vi "combined_broken.vi"() -> ()   [LabVIEW 2020]
uses:
  C:/Users/Public/Documents/Photometrics/PMQI-LabViewSamples/Examples/2018/Dependencies/PVCamNET.dll
  Dependencies/PVCamNET.dll
panel:
  out "SavingPath":string
  out "Saving":bool
  out "Capturing":bool
  in  "seq_save":bool
  in  "seq_start":bool
  in  "Path":path
  in  "FramesToCapture":u16=10
  in  "Full CCD Height":u16
  in  "Full CCD Width":u16
  in  "Full CCD":bool
  in  "Get ROI":bool
  in  "Height":u16
  in  "Y":u16
  in  "Width":u16
  in  "X":u16
  out "Trigger Mode":i32
  in  "Trigger In Behaviour":string(combo)="Edge Trigger"
  out "Exp. out":i32
  in  "Trigger Out Behaviour":string(combo)="Any Row"
  out "Boolean":bool
  in  "Scan Direction Reset":bool
  out "Scan Line Time":dbl format="%#_14g"
  in  "Scan Width":dbl=16.0
  in  "Scan Line Delay":dbl
  in  "Scan Direction":string(combo)="Up"
  in  "Scan Mode":string(combo)="Scan Width"
  in  "Exposure Time":dbl=5.0
  in  "Live":bool
  in  "Camera Status":bool
  in  "Uninit":bool
  in  "Live stop":bool
  in  "Live start":bool
  in  "Open":bool
  # "Description:\nThis interface can be used for both live imaging\nand sequence acquisition.\n\nSteps to run:\n1. Click the \"Run\" arrow\n2. Click \"Open\"\n3. Add desired parameters\n\nTo run live imaging: click \"Live Start\". If\nparameters need to be changed while imaging,\nfirst click \"Live Stop\" and then change\nparameters before starting again.\n\nTo execute sequence acquisition: click\n\"Sequence Start\". AFTER sequence has been\ncompleted (signified by the \"Capturing\" light\nturning off), click \"Sequence Save\" to save\nimages to desired folder.\n\n4. Click \"Close\" after finished imaging"
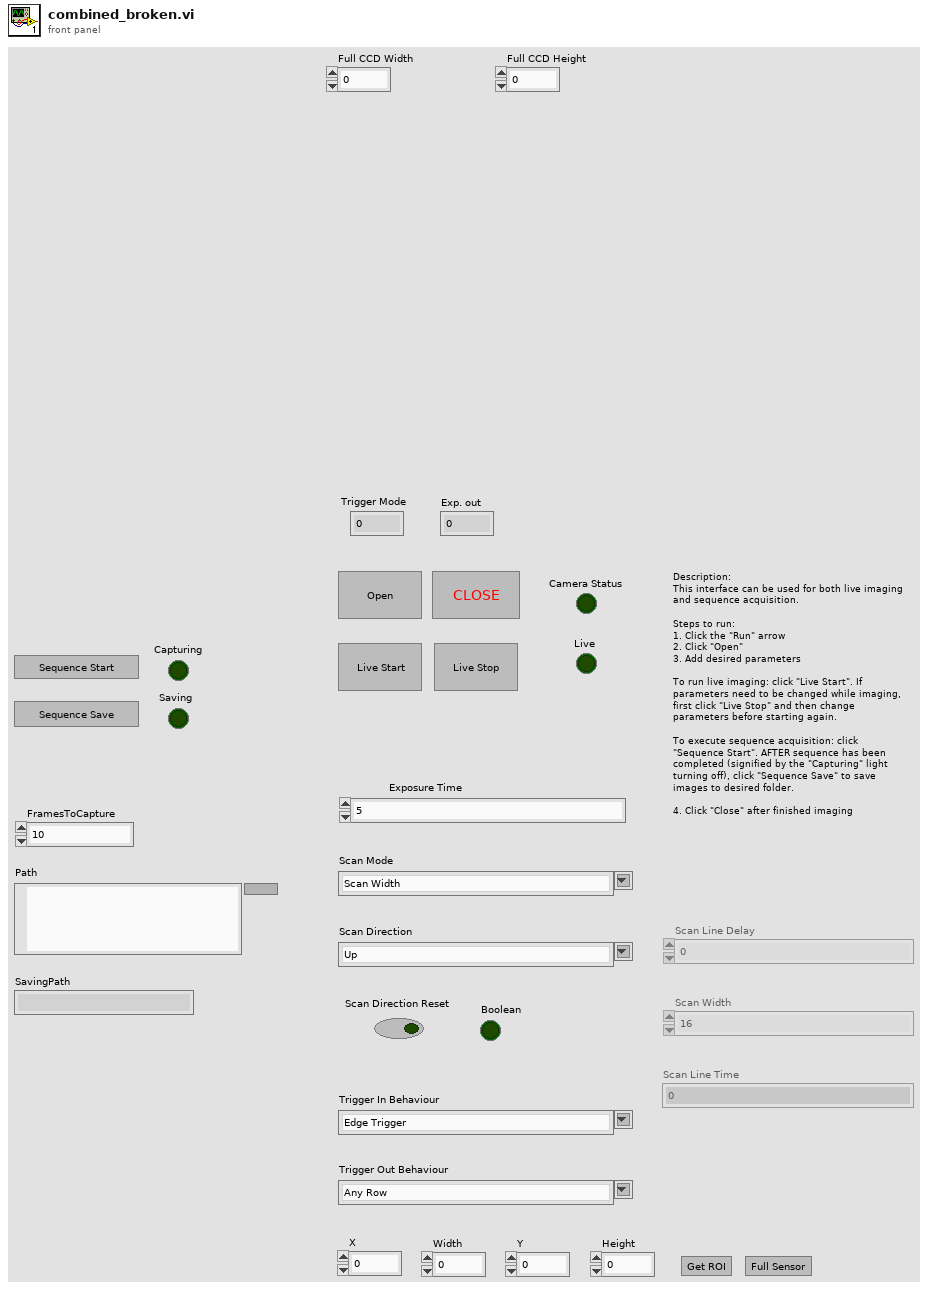
[diagram p1: front panel]
types:
  T1 = enum8{"Enabled", "Disabled", "Disabled and Grayed Out"}
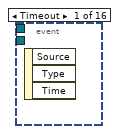
[diagram p2: hidden frame]
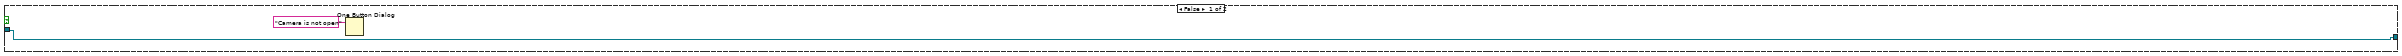
[diagram p15: hidden frame]
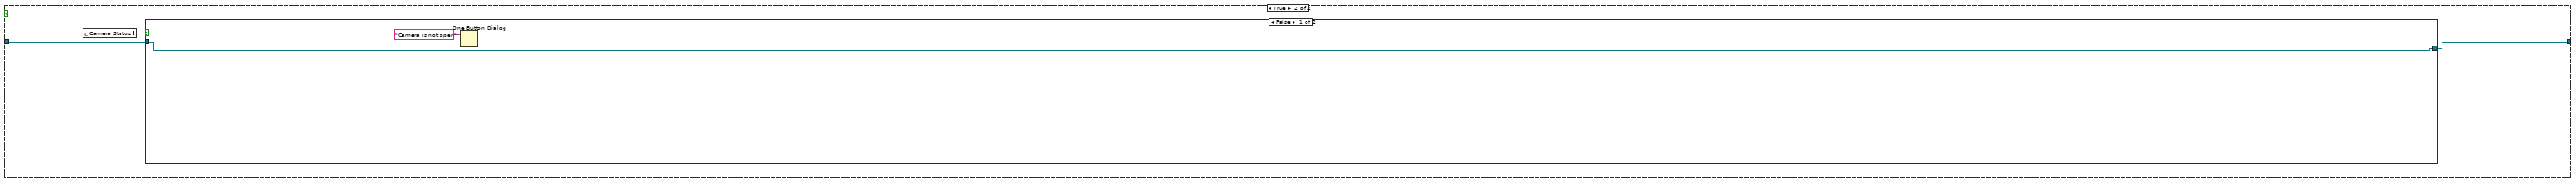
[diagram p18: hidden frame]
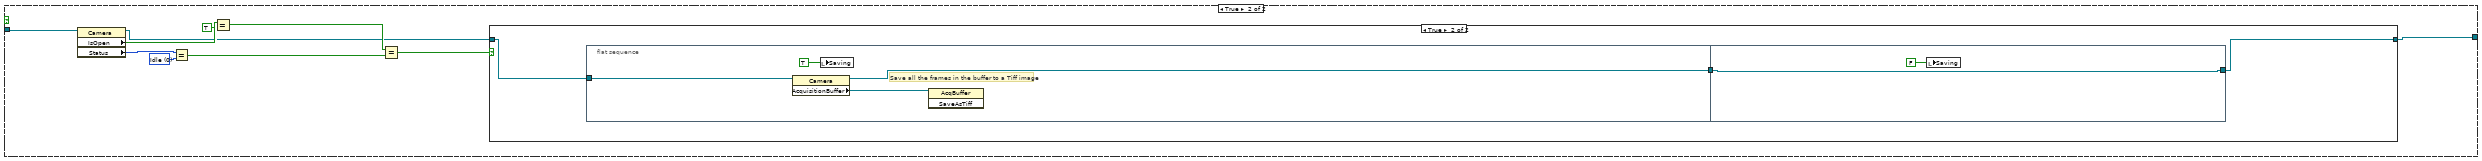
[diagram p19: hidden frame]
diagram:
  w16 = T1."Disabled and Grayed Out" ("Disabled")
  n1 = flat-sequence {
    tunnel: [w32] -> w31
    tunnel: w31 -> [w34]
    tunnel: [w33] -> w30
    tunnel: w30 -> [w874]
    frame #0 {
      n2 = property class="Library"() -> ("Instance"=w32:refnum<k24>)  [unwired: 2 in, 2 out]
    }
    frame #1 {
      n3 = while {
        tunnel: w34 -> [w39]
        shift-right: [w38] -> _
        shift-left: _ -> [w36]
        tunnel: [w37] -> w33
        stop <- w35 stop-if-true
        n4 = event shown="[1] \"Open\": Value Change" {
          selector: _ -> [_ _ _ _ _ _ _ _ _ _ _ _ _ _ _ _]
          dyn-events: _ -> [_ _ _ _ _ _ _ _ _ _ _ _ _ _ _ _]
          timeout: _ -> [_ _ _ _ _ _ _ _ _ _ _ _ _ _ _ _]
          tunnel: w39 -> [_ w44 _ _ _ _ _ _ w548 _ _ _ _ w791 _ w846]
          tunnel: [_ w43 w203 w234 w261 w293 w425 w489 w549 w616 w653 w726 w753 w792 w821 w847] -> w38
          tunnel: [_ w42 _ _ _ _ _ _ w548 _ _ _ _ w791 _ w846] -> w37
          tunnel: w36 -> [_ w41 w204 w233 w265 w294 w431 w491 w550 w617 w654 w727 w754 w793 w822 w848]
          tunnel: [_ _ _ _ _ _ _ _ _ _ _ _ _ _ _ w845] -> w35
          event Timeout {
            n5 = event-data() -> ()  [unwired: 1 in, 3 out]
          }
          event "Open": Value Change {
            n6 = event-data() -> ()  [unwired: 1 in, 6 out]
            n7 = case shown="True" "Open" {
              tunnel: w44 -> [w46 w52]
              tunnel: [w45 w51] -> w43
              tunnel: [w46 w50] -> w42
              tunnel: w41 -> [w45 w47]
              frame False {
              }
              frame True {
                n8 = local read "Camera Status"() -> (w49:bool)
                n9 = Not(x=w49) -> (.not. x?=w48:bool)
                n10 = case shown="True" w48 {
                  tunnel: w52 -> [w53 w59]
                  tunnel: [w54 w58] -> w51
                  tunnel: [w53 w57] -> w50
                  tunnel: w47 -> [w54 _]
                  frame False {
                  }
                  frame True {
                    n11 = flat-sequence {
                      tunnel: w59 -> [w64]
                      tunnel: [w66] -> w61
                      tunnel: [w65] -> w60
                      tunnel: w61 -> [w72]
                      tunnel: w60 -> [w73]
                      tunnel: [w73] -> w56
                      tunnel: [w71] -> w55
                      tunnel: [w116] -> w57
                      tunnel: [w96] -> w58
                      tunnel: w56 -> [w115]
                      tunnel: w55 -> [w116]
                      frame #0 {
                        # "Getting Camera at 0 index"
                        n12 = property class="Library"(reference=w64) -> ("Instance"=w63:refnum<k24>)  [unwired: 1 in, 2 out]
                        n13 = invoke class="Library" method="LoadCameras"(reference=w63) -> (reference out=w62:refnum<k24>)  [unwired: 2 in, 2 out]
                        n14 = property class="Library"(reference=w62) -> (reference out=w66:refnum<k24>, "Cameras"=w69:refnum<k24>)  [unwired: 1 in, 1 out]
                        n15 = invoke class="PmReadOnlyObservableCollection`" method="get_Item"(reference=w69, "index"=0) -> ("get_Item"=w67:refnum<k24>)  [unwired: 2 in, 3 out]
                        n16 = invoke class="Camera" method="Open"(reference=w67) -> (reference out=w65:refnum<k24>)  [unwired: 2 in, 2 out]
                      }
                      frame #1 {
                        n17 = invoke class="Library" method="ShowImage"(reference=w72, "cam"=w73) -> (reference out=w71:refnum<k24>)  [unwired: 2 in, 3 out]
                        n18 = local write "Camera Status"(TRUE ("Camera Status")) -> ()
                      }
                      frame #2 {
                        # "register callback"
                        n19 = property class="Camera"(reference=w115) -> (reference out=w97:refnum<k24>, "Settings"=w86:refnum<k24>)  [unwired: 1 in, 1 out]
                        n20 = property class="Camera"(reference=w97) -> (reference out=w96:refnum<k24>, "AcquisitionBuffer"=w95:refnum<k24>)  [unwired: 1 in, 1 out]
                        n21 = property class="CameraSettings"(reference=w86) -> ("ScanMode"=w114:refnum<k24>, "ScanDirection"=w110:refnum<k24>, "ScanLineDelay"=w105:refnum<k24>, "ScanWidth"=w92:refnum<k24>, "ScanLineTime"=w84:refnum<k24>, "ScanDirectionReset"=w100:refnum<k24>, "ExposeOutMode"=w88:refnum<k24>, "SensorHeight"=w79:refnum<k24>, "SensorWidth"=w78:refnum<k24>, "ExposureMode"=w74:refnum<k24>)  [unwired: 1 in, 2 out]
                        n22 = property class="PmEnumParam"(reference=w74) -> (reference out=w77:refnum<k24>, "Available"=w76:bool)  [unwired: 1 in, 1 out]
                        n23 = property class="PmNumericParam`1[[System.UInt32"(reference=w105) -> (reference out=w103:refnum<k24>, "Available"=w104:bool)  [unwired: 1 in, 1 out]
                        n24 = property class="PmNumericParam`1[[System.UInt32"(reference=w79) -> ("Max"=w81:u32)  [unwired: 1 in, 2 out]
                        n25 = property class="PmNumericParam`1[[System.UInt32"(reference=w78) -> ("Max"=w80:u32)  [unwired: 1 in, 2 out]
                        n26 = property class="PmNumericParam`1[[System.Int64,"(reference=w84) -> (reference out=w82:refnum<k24>, "Available"=w83:bool)  [unwired: 1 in, 1 out]
                        n27 = property class="PmNumericParam`1[[System.UInt32"(reference=w92) -> (reference out=w91:refnum<k24>, "Available"=w93:bool)  [unwired: 1 in, 1 out]
                        n28 = property class="AcqBuffer"(reference=w95, "UseScaling"=TRUE) -> ()  [unwired: 1 in, 2 out]
                        n29 = property class="PmEnumParam"(reference=w88) -> (reference out=w89:refnum<k24>, "Available"=w90:bool)  [unwired: 1 in, 1 out]
                        n30 = property class="PmEnumParam"(reference=w114) -> (reference out=w112:refnum<k24>, "Available"=w113:bool)  [unwired: 1 in, 1 out]
                        n31 = property class="PmEnumParam"(reference=w110) -> (reference out=w108:refnum<k24>, "Available"=w109:bool)  [unwired: 1 in, 1 out]
                        n32 = property class="PmBoolParam"(reference=w100) -> (reference out=w98:refnum<k24>, "Available"=w99:bool)  [unwired: 1 in, 1 out]
                        n33 = control-ref of="Trigger Out Behaviour"() -> (w87:refnum<vi>)
                        n34 = control-ref of="Scan Line Delay"() -> (w102:refnum<vi>)
                        n35 = control-ref of="Scan Line Time"() -> (w101:refnum<vi>)
                        n36 = control-ref of="Scan Mode"() -> (w111:refnum<vi>)
                        n37 = control-ref of="Scan Direction"() -> (w107:refnum<vi>)
                        n38 = control-ref of="Scan Width"() -> (w106:refnum<vi>)
                        n39 = control-ref of="Trigger In Behaviour"() -> (w75:refnum<vi>)
                        n40 = case shown="True" w99 {
                          tunnel: w98 -> [_ w148]
                          frame False {
                          }
                          frame True {
                            n41 = property class="PmBoolParam"(reference=w148) -> ("Current"=w147:bool)  [unwired: 1 in, 2 out]
                            n42 = local write "Scan Direction Reset"(w147) -> ()
                          }
                        }
                        n43 = case shown="True" w83 {
                          tunnel: w101 -> [_ w150]
                          tunnel: w82 -> [_ w149]
                          frame False {
                          }
                          frame True {
                            n44 = property class="PmNumericParam`1[[System.Int64,"(reference=w149) -> ("Max"=w151:i64, "Min"=w152:i64, "Current"=w153:i64)  [unwired: 1 in, 2 out]
                            n45 = In Range and Coerce(upper limit=w151, x=w153, lower limit=w152) -> (coerced(x)=w154:i64)  [unwired: 1 out]
                            n46 = property class="DigNum (strict)"(reference=w150, "Value"=w154) -> ()  [unwired: 1 in, 2 out]
                          }
                        }
                        n47 = case shown="True" w104 {
                          tunnel: w106 -> [_ w165]
                          tunnel: w103 -> [_ w164]
                          frame False {
                          }
                          frame True {
                            n48 = property class="PmNumericParam`1[[System.UInt32"(reference=w164) -> (reference out=w163:refnum<k24>, "Max"=w166:u32, "Min"=w167:u32, "Current"=w168:u32)  [unwired: 1 in, 1 out]
                            n49 = In Range and Coerce(upper limit=w166, x=w168, lower limit=w167) -> (coerced(x)=w162:u32)  [unwired: 1 out]
                            n50 = property class="PmNumericParam`1[[System.UInt32"(reference=w163, "Current"=w162) -> ()  [unwired: 1 in, 2 out]
                            n51 = property class="DigNum (strict)"(reference=w165, "Value"=w162) -> ()  [unwired: 1 in, 2 out]
                          }
                        }
                        n52 = case shown="True" w93 {
                          tunnel: w102 -> [_ w158]
                          tunnel: w91 -> [_ w157]
                          frame False {
                          }
                          frame True {
                            n53 = property class="PmNumericParam`1[[System.UInt32"(reference=w157) -> (reference out=w156:refnum<k24>, "Max"=w159:u32, "Min"=w160:u32, "Current"=w161:u32)  [unwired: 1 in, 1 out]
                            n54 = In Range and Coerce(upper limit=w159, x=w161, lower limit=w160) -> (coerced(x)=w155:u32)  [unwired: 1 out]
                            n55 = property class="PmNumericParam`1[[System.UInt32"(reference=w156, "Current"=w155) -> ()  [unwired: 1 in, 2 out]
                            n56 = property class="DigNum (strict)"(reference=w158, "Value"=w155) -> ()  [unwired: 1 in, 2 out]
                          }
                        }
                        n57 = case shown="True" w90 {
                          tunnel: w89 -> [_ w141]
                          tunnel: w87 -> [_ w132]
                          frame False {
                          }
                          frame True {
                            n58 = property class="PmEnumParam"(reference=w141) -> ("Options"=w140:refnum<k24>)  [unwired: 1 in, 2 out]
                            n59 = property class="PmReadOnlyObservableCollection`"(reference=w140) -> (reference out=w138:refnum<k24>, "Count"=w139:i32)  [unwired: 1 in, 1 out]
                            n60 = for {
                              N: w139 -> [_]
                              tunnel: w138 -> [w146]
                              tunnel: [w143] -> w135
                              tunnel: [w142] -> w134 mode=indexing
                              i -> [w145]
                              n61 = invoke class="PmReadOnlyObservableCollection`" method="get_Item"(reference=w146, "index"=w145) -> (reference out=w143:refnum<k24>, "get_Item"=w144:refnum<k24>)  [unwired: 2 in, 2 out]
                              n62 = property class="PmEnumItem"(reference=w144) -> ("Name"=w142:string)  [unwired: 1 in, 2 out]
                            }
                            n63 = invoke class="PmReadOnlyObservableCollection`" method="get_Item"(reference=w135, "index"=0) -> ("get_Item"=w136:refnum<k24>)  [unwired: 2 in, 3 out]
                            n64 = property class="PmEnumItem"(reference=w136) -> ("Name"=w133:string)  [unwired: 1 in, 2 out]
                            n65 = property class="CmbBox"(reference=w132, "Strings[]"=w134, "Value"=w133) -> ()  [unwired: 1 in, 2 out]
                          }
                        }
                        n66 = local write "Full CCD Height"(w81) -> ()
                        n67 = case shown="True" w113 {
                          tunnel: w112 -> [_ w197]
                          tunnel: w111 -> [_ w189]
                          frame False {
                          }
                          frame True {
                            n68 = property class="PmEnumParam"(reference=w197) -> (reference out=w188:refnum<k24>, "Options"=w196:refnum<k24>)  [unwired: 1 in, 1 out]
                            n69 = property class="PmReadOnlyObservableCollection`"(reference=w196) -> (reference out=w194:refnum<k24>, "Count"=w195:i32)  [unwired: 1 in, 1 out]
                            n70 = for {
                              N: w195 -> [_]
                              tunnel: w194 -> [w202]
                              tunnel: [w199] -> w192
                              tunnel: [w198] -> w191 mode=indexing
                              i -> [w201]
                              n71 = invoke class="PmReadOnlyObservableCollection`" method="get_Item"(reference=w202, "index"=w201) -> (reference out=w199:refnum<k24>, "get_Item"=w200:refnum<k24>)  [unwired: 2 in, 2 out]
                              n72 = property class="PmEnumItem"(reference=w200) -> ("Name"=w198:string)  [unwired: 1 in, 2 out]
                            }
                            n73 = invoke class="PmReadOnlyObservableCollection`" method="get_Item"(reference=w192, "index"=0) -> ("get_Item"=w187:refnum<k24>)  [unwired: 2 in, 3 out]
                            n74 = property class="PmEnumItem"(reference=w187) -> (reference out=w186:refnum<k24>, "Name"=w190:string)  [unwired: 1 in, 1 out]
                            n75 = property class="PmEnumParam"(reference=w188, "Current"=w186) -> ()  [unwired: 1 in, 2 out]
                            n76 = property class="CmbBox"(reference=w189, "Strings[]"=w191, "Value"=w190) -> ()  [unwired: 1 in, 2 out]
                          }
                        }
                        n77 = case shown="True" w109 {
                          tunnel: w108 -> [_ w180]
                          tunnel: w107 -> [_ w171]
                          frame False {
                          }
                          frame True {
                            n78 = property class="PmEnumParam"(reference=w180) -> (reference out=w170:refnum<k24>, "Options"=w179:refnum<k24>)  [unwired: 1 in, 1 out]
                            n79 = property class="PmReadOnlyObservableCollection`"(reference=w179) -> (reference out=w177:refnum<k24>, "Count"=w178:i32)  [unwired: 1 in, 1 out]
                            n80 = for {
                              N: w178 -> [_]
                              tunnel: w177 -> [w185]
                              tunnel: [w182] -> w174
                              tunnel: [w181] -> w173 mode=indexing
                              i -> [w184]
                              n81 = invoke class="PmReadOnlyObservableCollection`" method="get_Item"(reference=w185, "index"=w184) -> (reference out=w182:refnum<k24>, "get_Item"=w183:refnum<k24>)  [unwired: 2 in, 2 out]
                              n82 = property class="PmEnumItem"(reference=w183) -> ("Name"=w181:string)  [unwired: 1 in, 2 out]
                            }
                            n83 = invoke class="PmReadOnlyObservableCollection`" method="get_Item"(reference=w174, "index"=0) -> ("get_Item"=w175:refnum<k24>)  [unwired: 2 in, 3 out]
                            n84 = property class="PmEnumItem"(reference=w175) -> (reference out=w169:refnum<k24>, "Name"=w172:string)  [unwired: 1 in, 1 out]
                            n85 = property class="PmEnumParam"(reference=w170, "Current"=w169) -> ()  [unwired: 1 in, 2 out]
                            n86 = property class="CmbBox"(reference=w171, "Strings[]"=w173, "Value"=w172) -> ()  [unwired: 1 in, 2 out]
                          }
                        }
                        n87 = local write "Full CCD Width"(w80) -> ()
                        n88 = case shown="True" w76 {
                          tunnel: w77 -> [_ w126]
                          tunnel: w75 -> [_ w117]
                          frame False {
                          }
                          frame True {
                            n89 = property class="PmEnumParam"(reference=w126) -> ("Options"=w125:refnum<k24>)  [unwired: 1 in, 2 out]
                            n90 = property class="PmReadOnlyObservableCollection`"(reference=w125) -> (reference out=w123:refnum<k24>, "Count"=w124:i32)  [unwired: 1 in, 1 out]
                            n91 = for {
                              N: w124 -> [_]
                              tunnel: w123 -> [w131]
                              tunnel: [w128] -> w122
                              tunnel: [w127] -> w119 mode=indexing
                              i -> [w130]
                              n92 = invoke class="PmReadOnlyObservableCollection`" method="get_Item"(reference=w131, "index"=w130) -> (reference out=w128:refnum<k24>, "get_Item"=w129:refnum<k24>)  [unwired: 2 in, 2 out]
                              n93 = property class="PmEnumItem"(reference=w129) -> ("Name"=w127:string)  [unwired: 1 in, 2 out]
                            }
                            n94 = invoke class="PmReadOnlyObservableCollection`" method="get_Item"(reference=w122, "index"=0) -> ("get_Item"=w120:refnum<k24>)  [unwired: 2 in, 3 out]
                            n95 = property class="PmEnumItem"(reference=w120) -> ("Name"=w118:string)  [unwired: 1 in, 2 out]
                            n96 = property class="CmbBox"(reference=w117, "Strings[]"=w119, "Value"=w118) -> ()  [unwired: 1 in, 2 out]
                          }
                        }
                        n97 = local read "Exposure Time"() -> (w85:dbl)
                        n98 = property class="CameraSettings"(reference=w86, "Exposure"=w85) -> ()  [unwired: 1 in, 2 out]
                      }
                    }
                  }
                }
              }
            }
          }
          event "seq_start": Value Change {
            n99 = event-data() -> ()  [unwired: 1 in, 6 out]
            n100 = case shown="True" "seq_start" {
              tunnel: w204 -> [w206 w209]
              tunnel: [w206 w207] -> w203
              frame False {
              }
              frame True {
                n101 = local read "Camera Status"() -> (w208:bool)
                n102 = case shown="True" w208 {
                  tunnel: w209 -> [w210 w215]
                  tunnel: [w210 w212] -> w207
                  frame False {
                    n103 = One Button Dialog(message="Camera is not open") -> ()  [unwired: 1 in, 1 out]
                  }
                  frame True {
                    w220 = 0 items=["Idle", "Capturing"] ("Status")
                    n104 = property class="Camera"(reference=w215) -> (reference out=w214:refnum<k24>, "IsOpen"=w219:bool, "Status"=w221:i32)  [unwired: 1 in, 1 out]
                    n105 = Equal?(x=w221, y=w220) -> (x = y?=w216:bool)
                    n106 = Equal?(x=w219, y=TRUE) -> (x = y?=w217:bool)
                    n107 = Equal?(x=w217, y=w216) -> (x = y?=w213:bool)
                    n108 = case shown="True" w213 {
                      tunnel: w214 -> [w222 w225]
                      tunnel: [w222 w223] -> w212
                      frame False {
                      }
                      frame True {
                        n109 = flat-sequence {
                          tunnel: w225 -> [w227]
                          tunnel: [w226] -> w224
                          tunnel: [w231] -> w223
                          tunnel: w224 -> [w230]
                          frame #0 {
                            # "Register a callback to know the camera's state \n(eg. idle, capturing)"
                            n110 = property class="Camera" props=["Settings"](reference=w227) -> (reference out=w226:refnum<k24>)  [unwired: 1 in, 2 out]
                            n111 = control-ref of="Capturing"() -> (w228:refnum<vi>)
                            n112 = vi-ref "PropertyChangedEventCallbackForCameraState.vi"() -> ("vi reference"=w229:refnum<vi>)
                            n113 = node(w226, w229, w228) -> ()  [unwired: 2 in, 2 out]
                          }
                          frame #1 {
                            n114 = invoke class="Camera" method="StartSequence"(reference=w230) -> (reference out=w231:refnum<k24>)  [unwired: 2 in, 2 out]
                          }
                        }
                      }
                    }
                  }
                }
              }
            }
          }
          event "seq_save": Value Change {
            n115 = event-data() -> ()  [unwired: 1 in, 6 out]
            n116 = case shown="False" "seq_save" {
              tunnel: [w235 w237] -> w234
              tunnel: w233 -> [w235 w236]
              frame False {
              }
              frame True {
                n117 = local read "Camera Status"() -> (w238:bool)
                n118 = case shown="False" w238 {
                  tunnel: [w239 w242] -> w237
                  tunnel: w236 -> [w239 w241]
                  frame False {
                    n119 = One Button Dialog(message="Camera is not open") -> ()  [unwired: 1 in, 1 out]
                  }
                  frame True {
                    w249 = 0 items=["Idle", "Capturing"] ("Status")
                    n120 = property class="Camera"(reference=w241) -> (reference out=w244:refnum<k24>, "IsOpen"=w248:bool, "Status"=w250:i32)  [unwired: 1 in, 1 out]
                    n121 = Equal?(x=w250, y=w249) -> (x = y?=w245:bool)
                    n122 = Equal?(x=w248, y=TRUE) -> (x = y?=w246:bool)
                    n123 = Equal?(x=w246, y=w245) -> (x = y?=w243:bool)
                    n124 = case shown="True" w243 {
                      tunnel: w244 -> [w251 w254]
                      tunnel: [w251 w253] -> w242
                      frame False {
                      }
                      frame True {
                        n125 = flat-sequence {
                          tunnel: [w256] -> w252
                          tunnel: w254 -> [w255]
                          tunnel: [w259] -> w253
                          tunnel: w252 -> [w259]
                          frame #0 {
                            # "Save all the frames in the buffer to a Tiff image"
                            n126 = property class="Camera"(reference=w255) -> (reference out=w256:refnum<k24>, "AcquisitionBuffer"=w258:refnum<k24>)  [unwired: 1 in, 1 out]
                            n127 = local write "Saving"(TRUE ("Camera Status")) -> ()
                            n128 = invoke class="AcqBuffer" method="SaveAsTiff"(reference=w258) -> ()  [unwired: 2 in, 3 out]
                          }
                          frame #1 {
                            n129 = local write "Saving"(FALSE ("Camera Status")) -> ()
                          }
                        }
                      }
                    }
                  }
                }
              }
            }
          }
          event "Scan Direction": Value Change {
            w269 = 0 items=["Idle", "Capturing"] ("Status")
            n130 = event-data() -> ()  [unwired: 1 in, 6 out]
            n131 = property class="Camera"(reference=w265) -> (reference out=w262:refnum<k24>, "IsOpen"=w268:bool, "Status"=w270:i32)  [unwired: 1 in, 1 out]
            n132 = Equal?(x=w268, y=TRUE) -> (x = y?=w264:bool)
            n133 = Equal?(x=w270, y=w269) -> (x = y?=w266:bool)
            n134 = Equal?(x=w264, y=w266) -> (x = y?=w263:bool)
            n135 = case shown="True" w263 {
              tunnel: w262 -> [w271 w275]
              tunnel: [w271 w272] -> w261
              frame False {
              }
              frame True {
                n136 = property class="Camera"(reference=w275) -> (reference out=w272:refnum<k24>, "Settings"=w276:refnum<k24>)  [unwired: 1 in, 1 out]
                n137 = property class="CameraSettings"(reference=w276) -> ("ScanDirection"=w274:refnum<k24>)  [unwired: 1 in, 2 out]
                n138 = property class="PmEnumParam"(reference=w274) -> (reference out=w277:refnum<k24>, "Available"=w278:bool)  [unwired: 1 in, 1 out]
                n139 = control-ref of="Scan Mode"() -> (w273:refnum<vi>)
                n140 = case shown="True" w278 {
                  tunnel: w277 -> [_ w286]
                  tunnel: w273 -> [_ w279]
                  frame False {
                  }
                  frame True {
                    n141 = property class="CmbBox"(reference=w279) -> (reference out=w281:refnum<vi>, "Strings[]"=w287:string[])  [unwired: 1 in, 1 out]
                    n142 = property class="CmbBox"(reference=w281) -> ("Value"=w280:string)  [unwired: 1 in, 2 out]
                    n143 = while {
                      tunnel: w287 -> [w291] mode=indexing
                      tunnel: [w289] -> w284
                      tunnel: w280 -> [w288]
                      i -> [w289]
                      stop <- w290 stop-if-true
                      n144 = Equal?(x=w291, y=w288) -> (x = y?=w290:bool)
                    }
                    n145 = property class="PmEnumParam"(reference=w286) -> (reference out=w283:refnum<k24>, "Options"=w285:refnum<k24>)  [unwired: 1 in, 1 out]
                    n146 = invoke class="PmReadOnlyObservableCollection`" method="get_Item"(reference=w285, "index"=w284) -> ("get_Item"=w282:refnum<k24>)  [unwired: 2 in, 3 out]
                    n147 = property class="PmEnumParam"(reference=w283, "Current"=w282) -> ()  [unwired: 1 in, 2 out]
                  }
                }
              }
            }
          }
          event "Scan Mode", "Scan Direction Reset": Value Change {
            n148 = event-data() -> ()  [unwired: 1 in, 6 out]
            n149 = local read "Camera Status"() -> (w292:bool)
            n150 = case shown="True" w292 {
              tunnel: w294 -> [w295 w300]
              tunnel: [w295 w298] -> w293
              frame False {
                n151 = One Button Dialog(message="Camera is not open") -> ()  [unwired: 1 in, 1 out]
              }
              frame True {
                w305 = 0 items=["Idle", "Capturing"] ("Status")
                n152 = property class="Camera"(reference=w300) -> (reference out=w299:refnum<k24>, "IsOpen"=w304:bool, "Status"=w306:i32)  [unwired: 1 in, 1 out]
                n153 = Equal?(x=w304, y=TRUE) -> (x = y?=w302:bool)
                n154 = Equal?(x=w306, y=w305) -> (x = y?=w301:bool)
                n155 = Equal?(x=w302, y=w301) -> (x = y?=w297:bool)
                n156 = case shown="True" w297 {
                  tunnel: w299 -> [w307 w346]
                  tunnel: [w307 w341] -> w298
                  frame False {
                  }
                  frame True {
                    # "For Scan mode type if Auto is chosen then Scan Width and Scan Line Delay are not configurable.\nIf Line Delay is chosen then Scan Line is configurable, but Scan Width is not configurable.\nSimilarly if Scan Delay is chosen then Scan Line Delay is configurable, but Scan Width is not configurable."
                    n157 = property class="Camera"(reference=w346) -> (reference out=w341:refnum<k24>, "Settings"=w345:refnum<k24>)  [unwired: 1 in, 1 out]
                    n158 = property class="CameraSettings"(reference=w345) -> (error out=w338:errorcluster, "ScanMode"=w344:refnum<k24>, "ScanDirection"=w340:refnum<k24>, "ScanWidth"=w336:refnum<k24>, "ScanLineDelay"=w335:refnum<k24>, "ScanLineTime"=w324:refnum<k24>, "ScanDirectionReset"=w313:refnum<k24>)  [unwired: 1 in, 1 out]
                    n159 = property class="PmEnumParam"(reference=w344, error in=w338) -> (reference out=w342:refnum<k24>, error out=w339:errorcluster, "Available"=w343:bool)
                    n160 = control-ref of="Scan Mode"() -> (w337:refnum<vi>)
                    n161 = case shown="True" w343 {
                      tunnel: w342 -> [_ w419]
                      tunnel: w337 -> [_ w414]
                      tunnel: w339 -> [w407 w413]
                      tunnel: [w407 w408] -> w323
                      frame False {
                      }
                      frame True {
                        n162 = property class="CmbBox"(reference=w414) -> (reference out=w415:refnum<vi>, "Strings[]"=w420:string[])  [unwired: 1 in, 1 out]
                        n163 = property class="CmbBox"(reference=w415) -> ("Value"=w410:string)  [unwired: 1 in, 2 out]
                        n164 = while {
                          tunnel: w420 -> [w424] mode=indexing
                          tunnel: [w422] -> w417
                          tunnel: w410 -> [w421]
                          i -> [w422]
                          stop <- w423 stop-if-true
                          n165 = Equal?(x=w424, y=w421) -> (x = y?=w423:bool)
                        }
                        n166 = property class="PmEnumParam"(reference=w419, error in=w413) -> (reference out=w416:refnum<k24>, error out=w412:errorcluster, "Options"=w418:refnum<k24>)
                        n167 = invoke class="PmReadOnlyObservableCollection`" method="get_Item"(reference=w418, error in=w412, "index"=w417) -> (error out=w411:errorcluster, "get_Item"=w409:refnum<k24>)  [unwired: 1 in, 2 out]
                        n168 = property class="PmEnumParam" props=["Current", "IsReadOnly"](reference=w416, error in=w411, "Current"=w409) -> (error out=w408:errorcluster)  [unwired: 2 out]
                      }
                    }
                    n169 = property class="PmEnumParam"(reference=w340, error in=w323) -> (reference out=w332:refnum<k24>, error out=w326:errorcluster, "Available"=w333:bool)
                    n170 = control-ref of="Scan Direction"() -> (w334:refnum<vi>)
                    n171 = case shown="True" w333 {
                      tunnel: w332 -> [_ w401]
                      tunnel: w334 -> [_ w393]
                      tunnel: w326 -> [w385 w392]
                      tunnel: [w385 w386] -> w325
                      frame False {
                      }
                      frame True {
                        n172 = property class="PmEnumParam"(reference=w401, error in=w392) -> (reference out=w387:refnum<k24>, error out=w391:errorcluster, "Options"=w400:refnum<k24>)
                        n173 = property class="PmReadOnlyObservableCollection`"(reference=w400) -> (reference out=w398:refnum<k24>, "Count"=w399:i32)  [unwired: 1 in, 1 out]
                        n174 = for {
                          N: w399 -> [_]
                          tunnel: w398 -> [w406]
                          tunnel: [w403] -> w396
                          tunnel: [w402] -> w395 mode=indexing
                          i -> [w405]
                          n175 = invoke class="PmReadOnlyObservableCollection`" method="get_Item"(reference=w406, "index"=w405) -> (reference out=w403:refnum<k24>, "get_Item"=w404:refnum<k24>)  [unwired: 2 in, 2 out]
                          n176 = property class="PmEnumItem"(reference=w404) -> ("Name"=w402:string)  [unwired: 1 in, 2 out]
                        }
                        n177 = invoke class="PmReadOnlyObservableCollection`" method="get_Item"(reference=w396, error in=w391, "index"=0) -> (error out=w390:errorcluster, "get_Item"=w388:refnum<k24>)  [unwired: 1 in, 2 out]
                        n178 = property class="PmEnumParam"(reference=w387, "Current"=w388) -> ()  [unwired: 1 in, 2 out]
                        n179 = property class="PmEnumItem"(reference=w388, error in=w390) -> (error out=w389:errorcluster, "Name"=w394:string)  [unwired: 1 out]
                        n180 = property class="CmbBox"(reference=w393, error in=w389, "Strings[]"=w395, "Value"=w394) -> (error out=w386:errorcluster)  [unwired: 1 out]
                      }
                    }
                    n181 = property class="PmNumericParam`1[[System.UInt32"(reference=w336, error in=w325) -> (reference out=w329:refnum<k24>, error out=w328:errorcluster, "Available"=w330:bool)
                    n182 = control-ref of="Scan Width"() -> (w331:refnum<vi>)
                    n183 = case shown="True" w330 {
                      tunnel: w331 -> [_ w381]
                      tunnel: w329 -> [_ w378]
                      tunnel: w328 -> [w375 w380]
                      tunnel: [w375 w379] -> w327
                      frame False {
                      }
                      frame True {
                        n184 = property class="PmNumericParam`1[[System.UInt32"(reference=w378) -> ("Current"=w382:u32, "IsReadOnly"=w377:bool)  [unwired: 1 in, 2 out]
                        n185 = case shown="False" w377 {
                          tunnel: [T1."Enabled" ("Disabled") T1."Disabled and Grayed Out" ("Disabled")] -> w376
                          frame False {
                          }
                          frame True {
                          }
                        }
                        n186 = property class="DigNum (strict)"(reference=w381, error in=w380, "Value"=w382, "DisabledEnum"=w376) -> (error out=w379:errorcluster)  [unwired: 1 out]
                      }
                    }
                    n187 = property class="PmNumericParam`1[[System.UInt32"(reference=w335, error in=w327) -> (reference out=w320:refnum<k24>, error out=w314:errorcluster, "Available"=w321:bool)
                    n188 = control-ref of="Scan Line Delay"() -> (w315:refnum<vi>)
                    n189 = case shown="True" w321 {
                      tunnel: w315 -> [_ w371]
                      tunnel: w320 -> [_ w368]
                      tunnel: w314 -> [w365 w370]
                      tunnel: [w365 w369] -> w317
                      frame False {
                      }
                      frame True {
                        n190 = property class="PmNumericParam`1[[System.UInt32"(reference=w368) -> ("Current"=w372:u32, "IsReadOnly"=w367:bool)  [unwired: 1 in, 2 out]
                        n191 = case shown="False" w367 {
                          tunnel: [T1."Enabled" ("Disabled") T1."Disabled and Grayed Out" ("Disabled")] -> w366
                          frame False {
                          }
                          frame True {
                          }
                        }
                        n192 = property class="DigNum (strict)"(reference=w371, error in=w370, "Value"=w372, "DisabledEnum"=w366) -> (error out=w369:errorcluster)  [unwired: 1 out]
                      }
                    }
                    n193 = property class="PmNumericParam`1[[System.Int64,"(reference=w324, error in=w317) -> (reference out=w319:refnum<k24>, error out=w316:errorcluster, "Available"=w322:bool)
                    n194 = control-ref of="Scan Line Time"() -> (w318:refnum<vi>)
                    n195 = case shown="True" w322 {
                      tunnel: w318 -> [_ w361]
                      tunnel: w319 -> [_ w358]
                      tunnel: w316 -> [w355 w360]
                      tunnel: [w355 w359] -> w309
                      frame False {
                      }
                      frame True {
                        n196 = property class="PmNumericParam`1[[System.Int64,"(reference=w358) -> ("Current"=w362:i64, "IsReadOnly"=w357:bool)  [unwired: 1 in, 2 out]
                        n197 = case shown="False" w357 {
                          tunnel: [T1."Enabled" ("Disabled") T1."Disabled and Grayed Out" ("Disabled")] -> w356
                          frame False {
                          }
                          frame True {
                          }
                        }
                        n198 = property class="DigNum (strict)"(reference=w361, error in=w360, "Value"=w362, "DisabledEnum"=w356) -> (error out=w359:errorcluster)  [unwired: 1 out]
                      }
                    }
                    n199 = property class="PmBoolParam"(reference=w313, error in=w309) -> (reference out=w311:refnum<k24>, error out=w308:errorcluster, "Available"=w312:bool)
                    n200 = control-ref of="Scan Direction Reset"() -> (w310:refnum<vi>)
                    n201 = case shown="True" w312 {
                      tunnel: w311 -> [_ w352]
                      tunnel: w310 -> [_ w354]
                      tunnel: w308 -> [_ w349]
                      frame False {
                      }
                      frame True {
                        n202 = property class="Bool (strict)"(reference=w354, error in=w349) -> (error out=w348:errorcluster, "Value"=w353:bool)  [unwired: 1 out]
                        n203 = property class="PmBoolParam"(reference=w352, error in=w348, "Current"=w353) -> (reference out=w351:refnum<k24>, error out=w347:errorcluster)
                        n204 = property class="PmBoolParam"(reference=w351, error in=w347) -> ("Current"=w350:bool)  [unwired: 2 out]
                        n205 = local write "Boolean"(w350) -> ()
                      }
                    }
                  }
                }
              }
            }
          }
          event "Scan Line Delay": Value Change {
            w436 = 0 items=["Idle", "Capturing"] ("Status")
            n206 = event-data() -> ()  [unwired: 1 in, 6 out]
            n207 = property class="Camera"(reference=w431) -> (reference out=w430:refnum<k24>, "IsOpen"=w435:bool, "Status"=w437:i32)  [unwired: 1 in, 1 out]
            n208 = Equal?(x=w435, y=TRUE) -> (x = y?=w433:bool)
            n209 = Equal?(x=w437, y=w436) -> (x = y?=w432:bool)
            n210 = control-ref of="Scan Line Delay"() -> (w427:refnum<vi>)
            n211 = control-ref of="Scan Line Time"() -> (w426:refnum<vi>)
            n212 = control-ref of="Scan Width"() -> (w428:refnum<vi>)
            n213 = Equal?(x=w433, y=w432) -> (x = y?=w429:bool)
            n214 = case shown="True" w429 {
              tunnel: w430 -> [w438 w460]
              tunnel: [w438 w459] -> w425
              tunnel: w427 -> [_ w458]
              tunnel: w428 -> [_ w457]
              tunnel: w426 -> [_ w441]
              frame False {
              }
              frame True {
                n215 = property class="Camera"(reference=w460) -> (reference out=w459:refnum<k24>, "Settings"=w456:refnum<k24>)  [unwired: 1 in, 1 out]
                n216 = property class="CameraSettings"(reference=w456) -> (reference out=w446:refnum<k24>, error out=w452:errorcluster, "ScanLineDelay"=w455:refnum<k24>)  [unwired: 1 in]
                n217 = property class="PmNumericParam`1[[System.UInt32"(reference=w455, error in=w452) -> (reference out=w453:refnum<k24>, error out=w451:errorcluster, "Available"=w454:bool)
                n218 = case shown="True" w454 {
                  tunnel: w458 -> [_ w477]
                  tunnel: w453 -> [_ w476]
                  tunnel: w451 -> [w472 w475]
                  tunnel: [w472 w473] -> w447
                  frame False {
                  }
                  frame True {
                    n219 = property class="PmNumericParam`1[[System.UInt32"(reference=w476) -> (reference out=w480:refnum<k24>, "Max"=w478:u32, "Min"=w479:u32)  [unwired: 1 in, 1 out]
                    n220 = property class="DigNum (strict)"(reference=w477, error in=w475) -> (reference out=w484:refnum<vi>, error out=w474:errorcluster, "Value"=w483:dbl)
                    n221 = In Range and Coerce(upper limit=w478, x=w483, lower limit=w479) -> (coerced(x)=w482:dbl)  [unwired: 1 out]
                    n222 = property class="PmNumericParam`1[[System.UInt32"(reference=w480, "Current"=w482) -> (reference out=w481:refnum<k24>)  [unwired: 1 in, 1 out]
                    n223 = property class="PmNumericParam`1[[System.UInt32"(reference=w481) -> ("Current"=w485:u32)  [unwired: 1 in, 2 out]
                    n224 = property class="DigNum (strict)"(reference=w484, error in=w474, "Value"=w485) -> (error out=w473:errorcluster)  [unwired: 1 out]
                  }
                }
                n225 = property class="CameraSettings"(reference=w446) -> ("ScanWidth"=w445:refnum<k24>, "ScanLineTime"=w444:refnum<k24>)  [unwired: 1 in, 2 out]
                n226 = property class="PmNumericParam`1[[System.UInt32"(reference=w445, error in=w447) -> (reference out=w449:refnum<k24>, error out=w448:errorcluster, "Available"=w450:bool)
                n227 = case shown="True" w450 {
                  tunnel: w457 -> [_ w468]
                  tunnel: w449 -> [_ w471]
                  tunnel: w448 -> [w466 w469]
                  tunnel: [w466 w470] -> w440
                  frame False {
                  }
                  frame True {
                    n228 = property class="PmNumericParam`1[[System.UInt32"(reference=w471) -> ("Current"=w467:u32)  [unwired: 1 in, 2 out]
                    n229 = property class="DigNum (strict)"(reference=w468, error in=w469, "Value"=w467) -> (error out=w470:errorcluster)  [unwired: 1 out]
                  }
                }
                n230 = property class="PmNumericParam`1[[System.Int64,"(reference=w444, error in=w440) -> (reference out=w442:refnum<k24>, error out=w439:errorcluster, "Available"=w443:bool)
                n231 = case shown="True" w443 {
                  tunnel: w442 -> [_ w465]
                  tunnel: w441 -> [_ w463]
                  tunnel: w439 -> [_ w462]
                  frame False {
                  }
                  frame True {
                    n232 = property class="PmNumericParam`1[[System.Int64,"(reference=w465, error in=w462) -> (error out=w461:errorcluster, "Current"=w464:i64)  [unwired: 1 out]
                    n233 = property class="DigNum (strict)"(reference=w463, error in=w461, "Value"=w464) -> ()  [unwired: 2 out]
                  }
                }
              }
            }
          }
          event "Scan Width": Value Change {
            w497 = 0 items=["Idle", "Capturing"] ("Status")
            n234 = event-data() -> ()  [unwired: 1 in, 6 out]
            n235 = property class="Camera"(reference=w491) -> (reference out=w490:refnum<k24>, "IsOpen"=w496:bool, "Status"=w498:i32)  [unwired: 1 in, 1 out]
            n236 = Equal?(x=w496, y=TRUE) -> (x = y?=w494:bool)
            n237 = Equal?(x=w498, y=w497) -> (x = y?=w493:bool)
            n238 = control-ref of="Scan Line Delay"() -> (w487:refnum<vi>)
            n239 = control-ref of="Scan Line Time"() -> (w486:refnum<vi>)
            n240 = control-ref of="Scan Width"() -> (w488:refnum<vi>)
            n241 = Equal?(x=w494, y=w493) -> (x = y?=w492:bool)
            n242 = case shown="True" w492 {
              tunnel: w490 -> [w499 w521]
              tunnel: [w499 w520] -> w489
              tunnel: w488 -> [_ w519]
              tunnel: w487 -> [_ w518]
              tunnel: w486 -> [_ w503]
              frame False {
              }
              frame True {
                n243 = property class="Camera"(reference=w521) -> (reference out=w520:refnum<k24>, "Settings"=w517:refnum<k24>)  [unwired: 1 in, 1 out]
                n244 = property class="CameraSettings"(reference=w517) -> (reference out=w500:refnum<k24>, error out=w513:errorcluster, "ScanWidth"=w516:refnum<k24>)  [unwired: 1 in]
                n245 = property class="PmNumericParam`1[[System.UInt32"(reference=w516, error in=w513) -> (reference out=w514:refnum<k24>, error out=w512:errorcluster, "Available"=w515:bool)
                n246 = case shown="True" w515 {
                  tunnel: w519 -> [_ w538]
                  tunnel: w514 -> [_ w537]
                  tunnel: w512 -> [w533 w536]
                  tunnel: [w533 w534] -> w508
                  frame False {
                  }
                  frame True {
                    n247 = property class="PmNumericParam`1[[System.UInt32"(reference=w537) -> (reference out=w541:refnum<k24>, "Max"=w539:u32, "Min"=w540:u32)  [unwired: 1 in, 1 out]
                    n248 = property class="DigNum (strict)"(reference=w538, error in=w536) -> (reference out=w545:refnum<vi>, error out=w535:errorcluster, "Value"=w544:dbl)
                    n249 = In Range and Coerce(upper limit=w539, x=w544, lower limit=w540) -> (coerced(x)=w543:dbl)  [unwired: 1 out]
                    n250 = property class="PmNumericParam`1[[System.UInt32"(reference=w541, "Current"=w543) -> (reference out=w542:refnum<k24>)  [unwired: 1 in, 1 out]
                    n251 = property class="PmNumericParam`1[[System.UInt32"(reference=w542) -> ("Current"=w546:u32)  [unwired: 1 in, 2 out]
                    n252 = property class="DigNum (strict)"(reference=w545, error in=w535, "Value"=w546) -> (error out=w534:errorcluster)  [unwired: 1 out]
                  }
                }
                n253 = property class="CameraSettings"(reference=w500) -> ("ScanLineDelay"=w507:refnum<k24>, "ScanLineTime"=w506:refnum<k24>)  [unwired: 1 in, 2 out]
                n254 = property class="PmNumericParam`1[[System.UInt32"(reference=w507, error in=w508) -> (reference out=w510:refnum<k24>, error out=w509:errorcluster, "Available"=w511:bool)
                n255 = case shown="True" w511 {
                  tunnel: w518 -> [_ w529]
                  tunnel: w510 -> [_ w532]
                  tunnel: w509 -> [w527 w530]
                  tunnel: [w527 w531] -> w502
                  frame False {
                  }
                  frame True {
                    n256 = property class="PmNumericParam`1[[System.UInt32"(reference=w532) -> ("Current"=w528:u32)  [unwired: 1 in, 2 out]
                    n257 = property class="DigNum (strict)"(reference=w529, error in=w530, "Value"=w528) -> (error out=w531:errorcluster)  [unwired: 1 out]
                  }
                }
                n258 = property class="PmNumericParam`1[[System.Int64,"(reference=w506, error in=w502) -> (reference out=w504:refnum<k24>, error out=w501:errorcluster, "Available"=w505:bool)
                n259 = case shown="True" w505 {
                  tunnel: w504 -> [_ w526]
                  tunnel: w503 -> [_ w524]
                  tunnel: w501 -> [_ w523]
                  frame False {
                  }
                  frame True {
                    n260 = property class="PmNumericParam`1[[System.Int64,"(reference=w526, error in=w523) -> (error out=w522:errorcluster, "Current"=w525:i64)  [unwired: 1 out]
                    n261 = property class="DigNum (strict)"(reference=w524, error in=w522, "Value"=w525) -> ()  [unwired: 2 out]
                  }
                }
              }
            }
          }
          event "Trigger In Behaviour", "Trigger Out Behaviour": Value Change {
            n262 = event-data() -> ()  [unwired: 1 in, 6 out]
            n263 = local read "Camera Status"() -> (w547:bool)
            n264 = case shown="True" w547 {
              tunnel: w550 -> [w552 w556]
              tunnel: [w552 w553] -> w549
              frame False {
                n265 = One Button Dialog(message="Camera is not open") -> ()  [unwired: 1 in, 1 out]
              }
              frame True {
                w561 = 0 items=["Idle", "Capturing"] ("Status")
                n266 = property class="Camera"(reference=w556) -> (reference out=w554:refnum<k24>, "IsOpen"=w560:bool, "Status"=w562:i32)  [unwired: 1 in, 1 out]
                n267 = Equal?(x=w560, y=TRUE) -> (x = y?=w558:bool)
                n268 = Equal?(x=w562, y=w561) -> (x = y?=w557:bool)
                n269 = Equal?(x=w558, y=w557) -> (x = y?=w555:bool)
                n270 = case shown="True" w555 {
                  tunnel: w554 -> [w563 w585]
                  tunnel: [w563 w577] -> w553
                  frame False {
                  }
                  frame True {
                    n271 = property class="Camera"(reference=w585) -> (reference out=w577:refnum<k24>, "Settings"=w572:refnum<k24>)  [unwired: 1 in, 1 out]
                    n272 = property class="CameraSettings"(reference=w572) -> (reference out=w571:refnum<k24>, "ExposureTime"=w570:refnum<k24>, "ExposureMode"=w564:refnum<k24>, "ExposeOutMode"=w569:refnum<k24>)  [unwired: 1 in, 1 out]
                    n273 = property class="PmEnumParam"(reference=w569) -> (reference out=w575:refnum<k24>, "Available"=w576:bool)  [unwired: 1 in, 1 out]
                    n274 = property class="PmNumericParam`1[[System.UInt64"(reference=w570) -> (reference out=w582:refnum<k24>, "Max"=w584:u64, "Min"=w583:u64)  [unwired: 1 in, 1 out]
                    n275 = property class="PmEnumParam"(reference=w564) -> (reference out=w566:refnum<k24>, "Available"=w565:bool)  [unwired: 1 in, 1 out]
                    n276 = control-ref of="Trigger In Behaviour"() -> (w567:refnum<vi>)
                    n277 = local read "Exposure Time"() -> (w579:dbl)
                    n278 = control-ref of="Trigger Mode"() -> (w568:refnum<vi>)
                    n279 = case shown="True" w565 {
                      tunnel: w566 -> [_ w595]
                      tunnel: w568 -> [_ w589]
                      tunnel: w567 -> [_ w586]
                      frame False {
                      }
                      frame True {
                        n280 = property class="CmbBox"(reference=w586) -> (reference out=w588:refnum<vi>, "Strings[]"=w596:string[])  [unwired: 1 in, 1 out]
                        n281 = property class="CmbBox"(reference=w588) -> ("Value"=w587:string)  [unwired: 1 in, 2 out]
                        n282 = while {
                          tunnel: w596 -> [w600] mode=indexing
                          tunnel: [w598] -> w593
                          tunnel: w587 -> [w597]
                          i -> [w598]
                          stop <- w599 stop-if-true
                          n283 = Equal?(x=w600, y=w597) -> (x = y?=w599:bool)
                        }
                        n284 = property class="PmEnumParam"(reference=w595) -> (reference out=w592:refnum<k24>, "Options"=w594:refnum<k24>)  [unwired: 1 in, 1 out]
                        n285 = invoke class="PmReadOnlyObservableCollection`" method="get_Item"(reference=w594, "index"=w593) -> ("get_Item"=w591:refnum<k24>)  [unwired: 2 in, 3 out]
                        n286 = property class="PmEnumParam"(reference=w592, "Current"=w591) -> ()  [unwired: 1 in, 2 out]
                        n287 = property class="PmEnumItem"(reference=w591) -> ("Value"=w590:i32)  [unwired: 1 in, 2 out]
                        n288 = property class="DigNum (strict)"(reference=w589, "Value"=w590) -> ()  [unwired: 1 in, 2 out]
                      }
                    }
                    n289 = In Range and Coerce(upper limit=w584, x=w579, lower limit=w583) -> (coerced(x)=w580:dbl)  [unwired: 1 out]
                    n290 = control-ref of="Trigger Out Behaviour"() -> (w573:refnum<vi>)
                    n291 = property class="CameraSettings"(reference=w571, "Exposure"=w580) -> ()  [unwired: 1 in, 2 out]
                    n292 = control-ref of="Exp. out"() -> (w574:refnum<vi>)
                    n293 = property class="PmNumericParam`1[[System.UInt64"(reference=w582, "Current"=w580) -> (reference out=w581:refnum<k24>)  [unwired: 1 in, 1 out]
                    n294 = case shown="True" w576 {
                      tunnel: w575 -> [_ w610]
                      tunnel: w574 -> [_ w604]
                      tunnel: w573 -> [_ w601]
                      frame False {
                      }
                      frame True {
                        n295 = property class="CmbBox"(reference=w601) -> (reference out=w603:refnum<vi>, "Strings[]"=w611:string[])  [unwired: 1 in, 1 out]
                        n296 = property class="CmbBox"(reference=w603) -> ("Value"=w602:string)  [unwired: 1 in, 2 out]
                        n297 = while {
                          tunnel: w611 -> [w615] mode=indexing
                          tunnel: [w613] -> w608
                          tunnel: w602 -> [w612]
                          i -> [w613]
                          stop <- w614 stop-if-true
                          n298 = Equal?(x=w615, y=w612) -> (x = y?=w614:bool)
                        }
                        n299 = property class="PmEnumParam"(reference=w610) -> (reference out=w607:refnum<k24>, "Options"=w609:refnum<k24>)  [unwired: 1 in, 1 out]
                        n300 = invoke class="PmReadOnlyObservableCollection`" method="get_Item"(reference=w609, "index"=w608) -> ("get_Item"=w606:refnum<k24>)  [unwired: 2 in, 3 out]
                        n301 = property class="PmEnumParam"(reference=w607, "Current"=w606) -> ()  [unwired: 1 in, 2 out]
                        n302 = property class="PmEnumItem"(reference=w606) -> ("Value"=w605:i32)  [unwired: 1 in, 2 out]
                        n303 = property class="DigNum (strict)"(reference=w604, "Value"=w605) -> ()  [unwired: 1 in, 2 out]
                      }
                    }
                    n304 = property class="PmNumericParam`1[[System.UInt64"(reference=w581) -> ("Current"=w578:u64)  [unwired: 1 in, 2 out]
                    n305 = local write "Exposure Time"(w578) -> ()
                  }
                }
              }
            }
          }
          event "Get ROI": Value Change {
            n306 = event-data() -> ()  [unwired: 1 in, 6 out]
            n307 = case shown="True" "Get ROI" {
              tunnel: w617 -> [w619 w622]
              tunnel: [w619 w621] -> w616
              frame False {
              }
              frame True {
                n308 = local read "Camera Status"() -> (w620:bool)
                n309 = case shown="True" w620 {
                  tunnel: w622 -> [w624 w628]
                  tunnel: [w624 w625] -> w621
                  frame False {
                    n310 = One Button Dialog(message="Camera is not open") -> ()  [unwired: 1 in, 1 out]
                  }
                  frame True {
                    w633 = 0 items=["Idle", "Capturing"] ("Status")
                    n311 = property class="Camera"(reference=w628) -> (reference out=w627:refnum<k24>, "IsOpen"=w632:bool, "Status"=w634:i32)  [unwired: 1 in, 1 out]
                    n312 = Equal?(x=w634, y=w633) -> (x = y?=w629:bool)
                    n313 = Equal?(x=w632, y=TRUE) -> (x = y?=w630:bool)
                    n314 = Equal?(x=w630, y=w629) -> (x = y?=w626:bool)
                    n315 = case shown="True" w626 {
                      tunnel: w627 -> [w636 w644]
                      tunnel: [w636 w643] -> w625
                      frame False {
                        n316 = One Button Dialog(message="Camera must be idle.") -> ()  [unwired: 1 in, 1 out]
                      }
                      frame True {
                        n317 = property class="Camera"(reference=w644) -> (reference out=w643:refnum<k24>, "Settings"=w642:refnum<k24>)  [unwired: 1 in, 1 out]
                        n318 = property class="CameraSettings"(reference=w642) -> ("Regions"=w641:refnum<k24>)  [unwired: 1 in, 2 out]
                        n319 = property class="PmObservableCollection`1[[PVCam"(reference=w641) -> (reference out=w637:refnum<k24>, "Count"=w640:i32)  [unwired: 1 in, 1 out]
                        n320 = Greater?(x=w640, y=0) -> (0:w638:bool)
                        n321 = case shown="True" w638 {
                          tunnel: w637 -> [_ w646]
                          frame False {
                            n322 = One Button Dialog(message="ROI is not created.") -> ()  [unwired: 1 in, 1 out]
                          }
                          frame True {
                            n323 = invoke class="PmObservableCollection`1[[PVCam" method="get_Item"(reference=w646, "index"=0) -> ("get_Item"=w652:refnum<k24>)  [unwired: 2 in, 3 out]
                            n324 = property class="PmRegion"(reference=w652) -> ("Height"=w650:u16, "Width"=w649:u16, "X"=w648:u16, "Y"=w647:u16)  [unwired: 1 in, 2 out]
                            n325 = local write "Width"(w649) -> ()
                            n326 = local write "X"(w648) -> ()
                            n327 = local write "Y"(w647) -> ()
                            n328 = local write "Height"(w650) -> ()
                          }
                        }
                      }
                    }
                  }
                }
              }
            }
          }
          event "X", "Width", "Y", "Height": Value Change {
            n329 = event-data() -> ()  [unwired: 1 in, 6 out]
            n330 = local read "Camera Status"() -> (w655:bool)
            n331 = case shown="True" w655 {
              tunnel: w654 -> [w656 w659]
              tunnel: [w656 w657] -> w653
              frame False {
              }
              frame True {
                w665 = 0 items=["Idle", "Capturing"] ("Status")
                n332 = property class="Camera"(reference=w659) -> (reference out=w658:refnum<k24>, "IsOpen"=w664:bool, "Status"=w666:i32)  [unwired: 1 in, 1 out]
                n333 = Equal?(x=w664, y=TRUE) -> (x = y?=w662:bool)
                n334 = Equal?(x=w666, y=w665) -> (x = y?=w661:bool)
                n335 = Equal?(x=w662, y=w661) -> (x = y?=w660:bool)
                n336 = case shown="True" w660 {
                  tunnel: w658 -> [w667 w669]
                  tunnel: [w667 w668] -> w657
                  frame False {
                  }
                  frame True {
                    n337 = flat-sequence {
                      tunnel: w669 -> [w717]
                      tunnel: [w716] -> w668
                      frame #0 {
                        # "if (!( x >= 0\n            && (x+width) <= full_width\n            &&  0 < width \n            && y >= 0\n            && (y+height) <= full_height\n            && 0 < height ))\n        {\n           printf(\"Incorrect range for a ROI. \\n\");\n        }"
                        n338 = local read "Width"() -> (w685:u16)
                        n339 = local read "X"() -> (w686:u16)
                        n340 = Add(x=w686, y=w685) -> (x+y=w680:u16)
                        n341 = local read "Height"() -> (w683:u16)
                        n342 = local read "Y"() -> (w682:u16)
                        n343 = Add(x=w683, y=w682) -> (x+y=w678:u16)
                        n344 = local read "Full CCD Width"() -> (w681:u16)
                        n345 = local read "Width"() -> (w677:u16)
                        n346 = local read "Height"() -> (w674:u16)
                        n347 = Less Or Equal?(x=w680, y=w681) -> (x <= y?=w697:bool)
                        n348 = Less?(x=u16 0 ("y"), y=w677) -> (x < y?=w696:bool)
                        n349 = local read "Full CCD Height"() -> (w679:u16)
                        n350 = local read "X"() -> (w687:u16)
                        n351 = local read "Y"() -> (w684:u16)
                        n352 = Greater Or Equal?(x=w687, y=u16 0) -> (x >= y?=w698:bool)
                        n353 = Greater Or Equal?(x=w684, y=u16 0) -> (x >= y?=w695:bool)
                        n354 = Less Or Equal?(x=w678, y=w679) -> (x <= y?=w694:bool)
                        n355 = And(x=w698, y=w697) -> (x .and. y?=w692:bool)
                        n356 = And(x=w696, y=w695) -> (x .and. y?=w691:bool)
                        n357 = Less?(x=u16 0 ("y"), y=w674) -> (x < y?=w693:bool)
                        n358 = And(x=w692, y=w691) -> (x .and. y?=w690:bool)
                        n359 = And(x=w694, y=w693) -> (x .and. y?=w689:bool)
                        n360 = And(x=w690, y=w689) -> (x .and. y?=w688:bool)
                        n361 = case shown="False" w688 {
                          tunnel: [w702 w709] -> w673
                          tunnel: [u16 0 ("X") w708] -> w670
                          tunnel: [u16 0 ("Y") w707] -> w671
                          tunnel: [w703 w706] -> w672
                          frame False {
                            n362 = local read "Full CCD Height"() -> (w703:u16)
                            n363 = local read "Full CCD Width"() -> (w702:u16)
                            n364 = One Button Dialog(message="Wrong ROI ! Resetting to full CCD") -> ()  [unwired: 1 in, 1 out]
                          }
                          frame True {
                            n365 = local read "Height"() -> (w706:u16)
                            n366 = local read "Width"() -> (w709:u16)
                            n367 = local read "X"() -> (w708:u16)
                            n368 = local read "Y"() -> (w707:u16)
                          }
                        }
                        n369 = local write "Width"(w673) -> ()
                        n370 = local write "X"(w670) -> ()
                        n371 = local write "Y"(w671) -> ()
                        n372 = local write "Height"(w672) -> ()
                      }
                      frame #1 {
                        n373 = property class="Camera"(reference=w717) -> (reference out=w716:refnum<k24>, "Settings"=w715:refnum<k24>)  [unwired: 1 in, 1 out]
                        n374 = property class="CameraSettings"(reference=w715) -> ("Regions"=w714:refnum<k24>)  [unwired: 1 in, 2 out]
                        n375 = property class="PmObservableCollection`1[[PVCam"(reference=w714) -> (reference out=w710:refnum<k24>, "Count"=w713:i32)  [unwired: 1 in, 1 out]
                        n376 = Greater?(x=w713, y=0) -> (0:w711:bool)
                        n377 = case shown="True" w711 {
                          tunnel: w710 -> [_ w723]
                          frame False {
                            n378 = One Button Dialog(message="ROI is not created.") -> ()  [unwired: 1 in, 1 out]
                          }
                          frame True {
                            n379 = invoke class="PmObservableCollection`1[[PVCam" method="get_Item"(reference=w723, "index"=0) -> ("get_Item"=w725:refnum<k24>)  [unwired: 2 in, 3 out]
                            n380 = local read "Height"() -> (w722:u16)
                            n381 = local read "Width"() -> (w721:u16)
                            n382 = local read "X"() -> (w720:u16)
                            n383 = local read "Y"() -> (w719:u16)
                            n384 = property class="PmRegion"(reference=w725, "Height"=w722, "Width"=w721, "X"=w720, "Y"=w719) -> ()  [unwired: 1 in, 2 out]
                          }
                        }
                      }
                    }
                  }
                }
              }
            }
          }
          event "Path", "FramesToCapture": Value Change {
            n385 = event-data() -> ()  [unwired: 1 in, 6 out]
            n386 = local read "Camera Status"() -> (w728:bool)
            n387 = case shown="True" w728 {
              tunnel: w727 -> [w729 w732]
              tunnel: [w729 w730] -> w726
              frame False {
              }
              frame True {
                w738 = 0 items=["Idle", "Capturing"] ("Status")
                n388 = property class="Camera"(reference=w732) -> (reference out=w731:refnum<k24>, "IsOpen"=w737:bool, "Status"=w739:i32)  [unwired: 1 in, 1 out]
                n389 = Equal?(x=w737, y=TRUE) -> (x = y?=w735:bool)
                n390 = Equal?(x=w739, y=w738) -> (x = y?=w734:bool)
                n391 = Equal?(x=w735, y=w734) -> (x = y?=w733:bool)
                n392 = case shown="True" w733 {
                  tunnel: w731 -> [w740 w743]
                  tunnel: [w740 w742] -> w730
                  frame False {
                  }
                  frame True {
                    n393 = Path To String(path="Path") -> (string=w750:string)
                    n394 = property class="Camera"(reference=w743) -> (reference out=w742:refnum<k24>, "Settings"=w746:refnum<k24>, "AcquisitionBuffer"=w747:refnum<k24>)  [unwired: 1 in, 1 out]
                    n395 = Concatenate Strings(w750, "\\" ("string")) -> (w752:string)
                    "SavingPath" <- w752
                    n396 = property class="CameraSettings"(reference=w746, "FramesToCapture"="FramesToCapture") -> ()  [unwired: 1 in, 2 out]
                    n397 = property class="AcqBuffer"(reference=w747, "BufferSize"="FramesToCapture", "ImageSavingPath"=w752, "BigTiffRequired"=FALSE) -> (reference out=w748:refnum<k24>)  [unwired: 1 in, 1 out]
                    n398 = property class="AcqBuffer"(reference=w748) -> ("ImageSavingPath"=w749:string)  [unwired: 1 in, 2 out]
                    n399 = local write "SavingPath"(w749) -> ()
                  }
                }
              }
            }
          }
          event "Full CCD": Value Change {
            n400 = event-data() -> ()  [unwired: 1 in, 6 out]
            n401 = case shown="True" "Full CCD" {
              tunnel: w754 -> [w756 w759]
              tunnel: [w756 w758] -> w753
              frame False {
              }
              frame True {
                n402 = local read "Camera Status"() -> (w757:bool)
                n403 = case shown="True" w757 {
                  tunnel: w759 -> [w761 w765]
                  tunnel: [w761 w762] -> w758
                  frame False {
                    n404 = One Button Dialog(message="Camera is not open") -> ()  [unwired: 1 in, 1 out]
                  }
                  frame True {
                    w770 = 0 items=["Idle", "Capturing"] ("Status")
                    n405 = property class="Camera"(reference=w765) -> (reference out=w764:refnum<k24>, "IsOpen"=w769:bool, "Status"=w771:i32)  [unwired: 1 in, 1 out]
                    n406 = Equal?(x=w771, y=w770) -> (x = y?=w766:bool)
                    n407 = Equal?(x=w769, y=TRUE) -> (x = y?=w767:bool)
                    n408 = Equal?(x=w767, y=w766) -> (x = y?=w763:bool)
                    n409 = case shown="True" w763 {
                      tunnel: w764 -> [w772 w781]
                      tunnel: [w772 w780] -> w762
                      frame False {
                      }
                      frame True {
                        n410 = property class="Camera"(reference=w781) -> (reference out=w780:refnum<k24>, "Settings"=w779:refnum<k24>)  [unwired: 1 in, 1 out]
                        n411 = property class="CameraSettings"(reference=w779) -> (reference out=w773:refnum<k24>, "Regions"=w774:refnum<k24>)  [unwired: 1 in, 1 out]
                        n412 = property class="PmObservableCollection`1[[PVCam"(reference=w774) -> (reference out=w775:refnum<k24>, "Count"=w778:i32)  [unwired: 1 in, 1 out]
                        n413 = Greater?(x=w778, y=0) -> (0:w776:bool)
                        n414 = case shown="True" w776 {
                          tunnel: w775 -> [_ _]
                          tunnel: w774 -> [_ w790]
                          tunnel: w773 -> [_ w784]
                          frame False {
                          }
                          frame True {
                            n415 = invoke class="PmObservableCollection`1[[PVCam" method="RemoveAt"(reference=w790, "index"=0) -> ()  [unwired: 2 in, 4 out]
                            n416 = property class="CameraSettings"(reference=w784) -> ("SensorWidth"=w786:refnum<k24>)  [unwired: 1 in, 2 out]
                            n417 = property class="CameraSettings"(reference=w784) -> ("SensorHeight"=w787:refnum<k24>)  [unwired: 1 in, 2 out]
                            n418 = property class="PmNumericParam`1[[System.UInt32"(reference=w786) -> ("Current"=w785:u32)  [unwired: 1 in, 2 out]
                            n419 = property class="PmNumericParam`1[[System.UInt32"(reference=w787) -> ("Current"=w788:u32)  [unwired: 1 in, 2 out]
                            n420 = local write "Width"(w785) -> ()
                            n421 = local write "Height"(w788) -> ()
                            n422 = local write "X"(0 ("index")) -> ()
                            n423 = local write "Y"(0 ("index")) -> ()
                          }
                        }
                      }
                    }
                  }
                }
              }
            }
          }
          event "Live start": Value Change {
            n424 = event-data() -> ()  [unwired: 1 in, 6 out]
            n425 = case shown="True" "Live start" {
              tunnel: w793 -> [w795 w798]
              tunnel: [w795 w797] -> w792
              frame False {
              }
              frame True {
                n426 = local read "Camera Status"() -> (w796:bool)
                n427 = case shown="True" w796 {
                  tunnel: w798 -> [w799 w804]
                  tunnel: [w799 w802] -> w797
                  frame False {
                    n428 = One Button Dialog(message="Camera is not open") -> ()  [unwired: 1 in, 1 out]
                  }
                  frame True {
                    w809 = 0 items=["Idle", "Capturing"] ("Status")
                    n429 = property class="Camera"(reference=w804) -> (reference out=w803:refnum<k24>, "IsOpen"=w808:bool, "Status"=w810:i32)  [unwired: 1 in, 1 out]
                    n430 = Equal?(x=w810, y=w809) -> (x = y?=w805:bool)
                    n431 = Equal?(x=w808, y=TRUE) -> (x = y?=w806:bool)
                    n432 = Equal?(x=w806, y=w805) -> (x = y?=w801:bool)
                    n433 = case shown="True" w801 {
                      tunnel: w803 -> [w812 w814]
                      tunnel: [w812 w815] -> w802
                      frame False {
                        n434 = local write "Live"(FALSE ("Live 2")) -> ()
                      }
                      frame True {
                        n435 = flat-sequence {
                          tunnel: w814 -> [w820]
                          tunnel: [w817] -> w813
                          frame #0 {
                            n436 = property class="Camera"(reference=w820) -> (reference out=w817:refnum<k24>, "AcquisitionBuffer"=w819:refnum<k24>)  [unwired: 1 in, 1 out]
                            n437 = property class="AcqBuffer"(reference=w819, "BufferSize"=100) -> ()  [unwired: 1 in, 2 out]
                          }
                        }
                        n438 = local write "Live"(TRUE ("Live")) -> ()
                        n439 = invoke class="Camera" method="StartLive"(reference=w813) -> (reference out=w815:refnum<k24>)  [unwired: 2 in, 2 out]
                      }
                    }
                  }
                }
              }
            }
          }
          event "Live stop": Value Change {
            n440 = event-data() -> ()  [unwired: 1 in, 6 out]
            n441 = case shown="True" "Live stop" {
              tunnel: w822 -> [w824 w827]
              tunnel: [w824 w826] -> w821
              frame False {
              }
              frame True {
                n442 = local read "Camera Status"() -> (w825:bool)
                n443 = case shown="False" w825 {
                  tunnel: w827 -> [w829 w839]
                  tunnel: [w829 w836] -> w826
                  frame False {
                    n444 = One Button Dialog(message="Camera is not open") -> ()  [unwired: 1 in, 1 out]
                  }
                  frame True {
                    w834 = 1 items=["Idle", "Capturing"] ("Status")
                    n445 = property class="Camera"(reference=w839) -> (reference out=w837:refnum<k24>, "IsOpen"=w833:bool, "Status"=w835:i32)  [unwired: 1 in, 1 out]
                    n446 = Equal?(x=w835, y=w834) -> (x = y?=w830:bool)
                    n447 = Equal?(x=w833, y=TRUE) -> (x = y?=w831:bool)
                    n448 = Equal?(x=w831, y=w830) -> (x = y?=w838:bool)
                    n449 = case shown="True" w838 {
                      tunnel: w837 -> [w840 w843]
                      tunnel: [w840 w842] -> w836
                      frame False {
                      }
                      frame True {
                        n450 = invoke class="Camera" method="Stop"(reference=w843) -> (reference out=w842:refnum<k24>)  [unwired: 2 in, 2 out]
                        n451 = local write "Live"(FALSE ("Live 2")) -> ()
                      }
                    }
                  }
                }
              }
            }
          }
          event "Uninit": Value Change {
            n452 = event-data() -> ()  [unwired: 1 in, 6 out]
            n453 = case shown="True" "Uninit" {
              tunnel: w848 -> [w850 w854]
              tunnel: [w850 w853] -> w847
              tunnel: [FALSE ("Camera Status") w851] -> w845
              frame False {
              }
              frame True {
                n454 = local read "Camera Status"() -> (w852:bool)
                n455 = case shown="True" w852 {
                  tunnel: w854 -> [w856 w861]
                  tunnel: [w856 w860] -> w853
                  tunnel: [FALSE ("Camera Status") w859] -> w851
                  frame False {
                  }
                  frame True {
                    n456 = local read "Live"() -> (w857:bool)
                    n457 = Not(x=w857) -> (.not. x?=w858:bool)
                    n458 = case shown="True" w858 {
                      tunnel: w861 -> [w863 w866]
                      tunnel: [w863 w865] -> w860
                      tunnel: [FALSE ("Camera Status") w864] -> w859
                      frame False {
                      }
                      frame True {
                        n459 = flat-sequence {
                          tunnel: w866 -> [w869]
                          tunnel: [w868] -> w867
                          tunnel: [w872] -> w865
                          tunnel: w867 -> [w872]
                          tunnel: [TRUE ("Camera Status")] -> w864
                          frame #0 {
                            n460 = invoke class="Camera" method="Close"(reference=w869) -> (reference out=w868:refnum<k24>)  [unwired: 2 in, 2 out]
                          }
                          frame #1 {
                            n461 = local write "Camera Status"(FALSE ("Camera Status")) -> ()
                          }
                        }
                      }
                    }
                  }
                }
              }
            }
          }
        }
      }
    }
    frame #2 {
      n462 = invoke class="Library" method="Release"(reference=w874) -> (reference out=w875:refnum<k24>)  [unwired: 2 in, 2 out]
      n463 = Wait (ms)(milliseconds to wait=u32 100) -> ()  [unwired: 1 out]
      n464 = Close Reference(reference=w875) -> ()  [unwired: 1 in, 1 out]
    }
    frame #3 {
      n465 = invoke class="GC" method="Collect"() -> ()  [unwired: 3 in, 3 out]
    }
  }
  n466 = local write "Camera Status"(FALSE ("Camera Status")) -> ()
  n467 = control-ref of="FramesToCapture"() -> (w5:refnum<vi>)
  n468 = property class="DigNum (strict)"(reference=w5, "Value"=10) -> ()  [unwired: 1 in, 2 out]
  n469 = control-ref of="Path"() -> (w3:refnum<vi>)
  n470 = String To Path(string="") -> (path=w1:path)
  n471 = property class="Path"(reference=w3, "Value"=w1) -> ()  [unwired: 1 in, 2 out]
  n472 = control-ref of="Scan Mode"() -> (w28:refnum<vi>)
  n473 = control-ref of="Scan Direction"() -> (w25:refnum<vi>)
  n474 = property class="CmbBox"(reference=w28, "Value"="", "Strings[]"=string[] [] ("Strings []")) -> ()  [unwired: 1 in, 2 out]
  n475 = property class="CmbBox"(reference=w25, "Strings[]"=string[] [] ("Strings []"), "Value"="") -> ()  [unwired: 1 in, 2 out]
  n476 = control-ref of="Trigger Mode"() -> (w7:refnum<vi>)
  n477 = control-ref of="Scan Line Delay"() -> (w19:refnum<vi>)
  n478 = control-ref of="Scan Line Time"() -> (w18:refnum<vi>)
  n479 = control-ref of="Exp. out"() -> (w8:refnum<vi>)
  n480 = control-ref of="Scan Width"() -> (w22:refnum<vi>)
  n481 = control-ref of="Exp. out"() -> (w11:refnum<vi>)
  n482 = property class="DigNum (strict)"(reference=w8, "Visible"=TRUE) -> ()  [unwired: 1 in, 2 out]
  n483 = property class="DigNum (strict)"(reference=w22, "Value"=0.0) -> ()  [unwired: 1 in, 2 out]
  n484 = property class="DigNum (strict)"(reference=w7, "Visible"=TRUE) -> ()  [unwired: 1 in, 2 out]
  n485 = property class="DigNum (strict)"(reference=w11, "Value"=0) -> ()  [unwired: 1 in, 2 out]
  n486 = property class="DigNum (strict)"(reference=w18, "Value"=0.0) -> ()  [unwired: 1 in, 2 out]
  n487 = property class="DigNum (strict)"(reference=w19, "Value"=0.0) -> ()  [unwired: 1 in, 2 out]
  n488 = property on="Scan Width" class="DigNum (strict)"("DisabledEnum"=w16) -> ()  [unwired: 2 in, 2 out]
  n489 = property on="Scan Line Delay" class="DigNum (strict)"("DisabledEnum"=w16) -> ()  [unwired: 2 in, 2 out]
  n490 = local write "Scan Direction Reset"(FALSE ("Boolean")) -> ()
  n491 = control-ref of="Trigger Out Behaviour"() -> (w13:refnum<vi>)
  n492 = property class="CmbBox"(reference=w13, "Value"="") -> ()  [unwired: 1 in, 2 out]
  "Boolean" <- FALSE ("Boolean")
